vi "RTM - Add Buffered Packet.vi"(8 "error in (no error)":errorcluster, 11 "Node Ptr":u64 format="%.0x") -> (0 "error out":errorcluster)   [LabVIEW 2019]
panel:
  in  "Cancel Button":bool
  in  "OK Button":bool
  out "New Packet ID":i32
  in  "New Packet Name":string
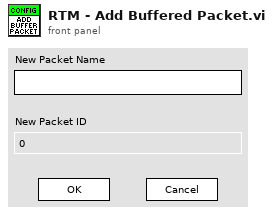
[diagram p1: front panel]
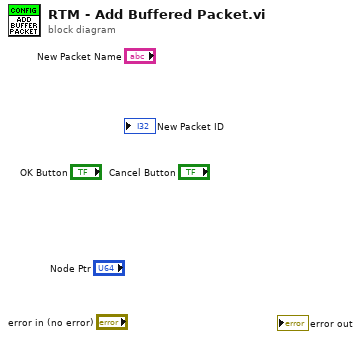
[diagram p0: block diagram]
diagram:
